vi "SPC_stream_stop_condition.vi"(5 "Stop OR Mask":u32 format="%x", 6 "Stream Handle":i16, 7 "Stop AND Mask":u32 format="%x", 8 "Error In":errorcluster, 9 "Stop Time":dbl, 11 "DLL Path":path) -> (0 "Error Out":errorcluster, 3 "DLL Path":path, 4 "Stream Handle":i16)   [LabVIEW 2023]
doc: "-stop_time: macro time (in sec) at which extracting photons will stop ( during call to SPC_get_photons_from_stream) (if stop masks are not defined) \n-stop_OR_mask: bitwise OR mask used to define stop of extracting photons from the stream ( in addition to 'stop_time'), bits 31-28 - markers M3-M0, bits 27-0 - routing channels 27-0 \n-stop_AND_mask bitwise AND mask used to define stop of extracting photons from the stream ( in addition to 'stop_time'), bits 31-28 - markers M3-M0, bits 27-0 - routing channels 27-0 \n\nThe procedure is used to define stop of extracting photons from buffered stream 'stream_hndl' during SPC_get_photons_from_stream call. \nStop_time and OR/AND masks can be used all together.\nAll photons (markers) are extracted until the macro time in the stream reaches 'stop_time' value. \nFrom this moment appearance of specified markers/channels is tested according to stop_OR(AND)_mask. \nStop condition is found when minimum one of markers/channels defined in stop_OR_mask appears in the stream (since 'stop_time').\nStop condition is also found when all of markers/channels defined in stop_AND_mask appeared in the stream (since 'stop_time').\nSPC_get_photons_from_stream returns an error, when stop condition cannot be found in the stream. \nWhile extracting photons during running measurement, stop condition (if defined) can be found later after reading new portion of photons data from FIFO to the stream (using SPC_read_fifo_to_stream). \n\ninfo@becker-hickl.com"
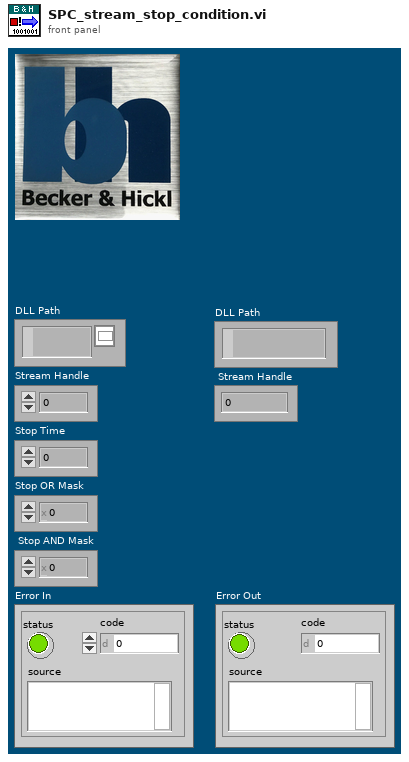
[diagram p1: front panel]
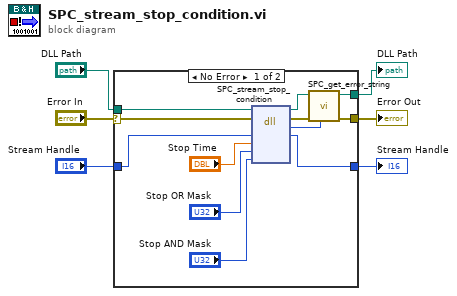
[diagram p0: block diagram]
diagram:
  n1 = case shown="No Error" "Error In" {
    selector: "Error In" -> [w14 w21]
    tunnel: "DLL Path" -> [w15 w20]
    tunnel: [w10 w20] -> w5
    tunnel: [w9 w21] -> w4
    tunnel: "Stream Handle" -> [w8 w19]
    tunnel: [w7 w19] -> w1
    frame No Error {
      n2 = dll-call lib="D:/spcm/lib/lab_view/lv10.0/spcm32.dll" fn="SPC_stream_stop_condition"(path in=w15, error in=w14, "stream_hndl"=w8, "stop_time"="Stop Time", "stop_OR_mask"="Stop OR Mask", "stop_AND_mask"="Stop AND Mask") -> (path out=w11:path, error out=w13:errorcluster, "return type"=w12:i16, "stream_hndl"=w7:i16)  [unwired: 4 in]
      n3 = call "SPC_get_error_string.vi"("ErrorID"=w12, "Error In"=w13, "DLL Path"=w11) -> ("Error Out"=w9:errorcluster, "DLL Path"=w10:path)  [unwired: 6 in, 1 out]
    }
    frame Error {
    }
  }
  "DLL Path" <- w5
  "Error Out" <- w4
  "Stream Handle" <- w1
